vi "CAlex2_SetLegDH.vi"(8 "error in (no error)":errorcluster, 9 "End Effector Pos":T1={"Coord4"=[0.0, 0.0, 0.0, 1.0], "ID"=4}, 10 "ArmProperty":T2, 11 "CAlex2 in":refnum<class "CAlex2.lvclass">) -> (0 "error out":errorcluster, 3 "CAlex2 out":refnum<class "CAlex2.lvclass">)   [LabVIEW 2016, in "CAlex2.lvclass"]
uses:
  CAlex2.lvclass
  C:/Users/randh/Desktop/CABLE-LABVIEW/CALEX/CAlex2-controller/Classes/SerialChain/SerialChain.lvclass
  TypeDef/LowerBodyDim.ctl
  SerialChain/TypeDef/PointOnBody.ctl
  SerialChain/TypeDef/xyzO.ctl
  SerialChain/TypeDef/JointType.ctl
  SerialChain/SerialChain.lvclass
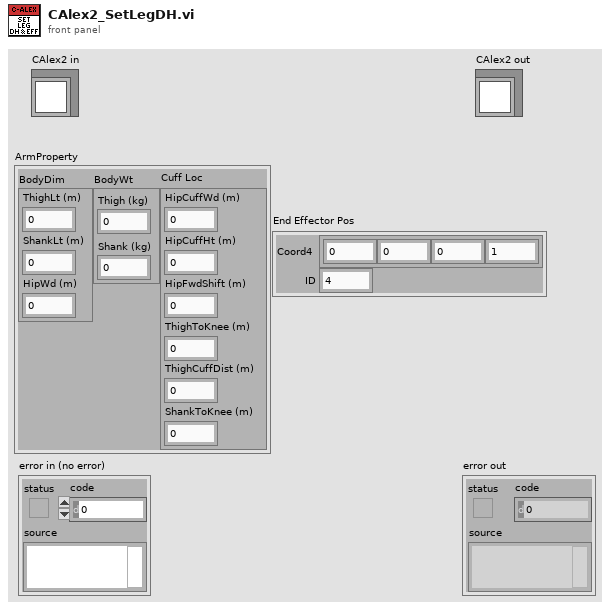
[diagram p1: front panel]
types:
  T1 = typedef "SerialChain.lvclass/PointOnBody.ctl" = cluster{"Coord4":dbl[], "ID":i32}
  T2 = typedef "CAlex2.lvclass/LowerBodyDim.ctl" = cluster{"BodyDim":cluster{"ThighLt (m)":dbl, "ShankLt (m)":dbl, "HipWd (m)":dbl}, "BodyWt":cluster{"Thigh (kg)":dbl, "Shank (kg)":dbl}, "Cuff Loc":cluster{"HipCuffWd (m)":dbl, "HipCuffHt (m)":dbl, "HipFwdShift (m)":dbl, "ThighToKnee (m)":dbl, "ThighCuffDist (m)":dbl, "ShankToKnee (m)":dbl}}
  T3 = typedef "SerialChain.lvclass/JointType.ctl" = enum16{"theta(hinge)", "alpha", "a", "d(slide)"}
  T4 = typedef "SerialChain.lvclass/xyzO.ctl" = enum16{"X", "Y", "Z", "O"}
  T5 = typedef "SerialChain.lvclass/DH_param.ctl" = cluster{"a":dbl, "d":dbl, "theta":dbl, "alpha":dbl, "JointType":T3}
  T6 = cluster{"DH Parameters":T5, "CoM_Pos":T1, "Mass(kg)":dbl}
  T7 = cluster{"DH Parameters":T5, "CoM_Pos":T1, "Mass(kg)":dbl}[]
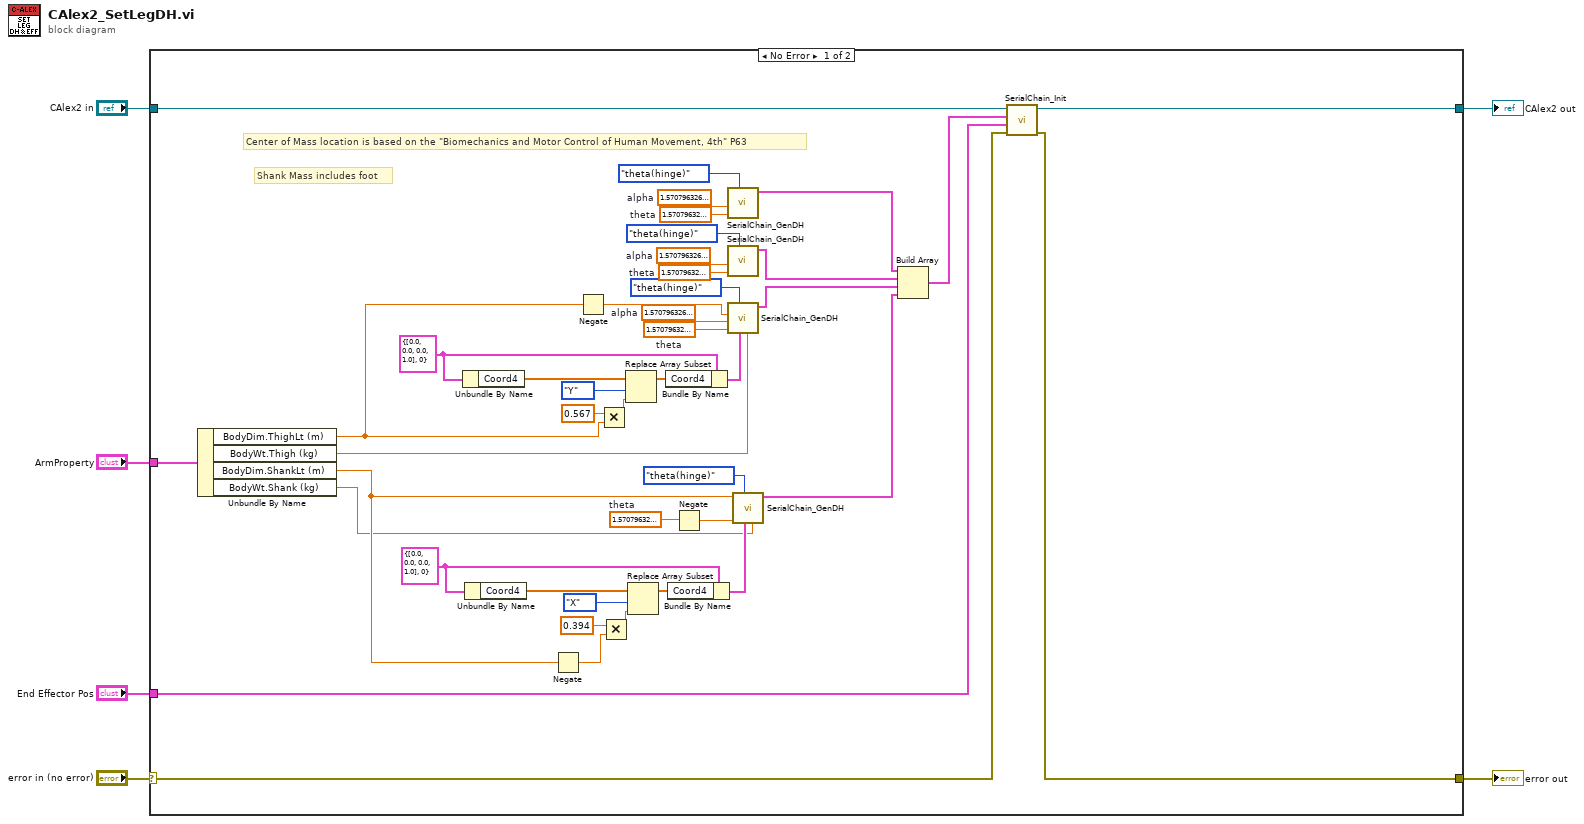
[diagram p0: block diagram]
diagram:
  n1 = case shown="No Error" "error in (no error)" {
    selector: "error in (no error)" -> [w17 w51]
    tunnel: [w8 w51] -> w5
    tunnel: [w7 w50] -> w3
    tunnel: "CAlex2 in" -> [w18 w50]
    tunnel: "ArmProperty" -> [w12 _]
    tunnel: "End Effector Pos" -> [w9 _]
    frame No Error {
      w21 = T1 {"Coord4"=[0.0, 0.0, 0.0, 1.0], "ID"=0} ("CoM_Pos")
      w31 = T1 {"Coord4"=[0.0, 0.0, 0.0, 1.0], "ID"=0} ("CoM_Pos")
      w38 = 1.5707963267948966  # theta
      w39 = 1.5707963267948966  # theta
      w40 = 1.5707963267948966  # theta
      w41 = 1.5707963267948966  # theta
      w48 = 1.5707963267948966  # alpha
      w42 = 1.5707963267948966  # alpha
      w49 = 1.5707963267948966  # alpha
      # "Shank Mass includes foot"
      # "Center of Mass location is based on the \"Biomechanics and Motor Control of Human Movement, 4th\" P63"
      n2 = Unbundle By Name(w12) -> ("BodyDim.ThighLt (m)"=w23:dbl, "BodyWt.Thigh (kg)"=w36:dbl, "BodyDim.ShankLt (m)"=w11:dbl, "BodyWt.Shank (kg)"=w10:dbl)
      n3 = Unbundle By Name(w31) -> ("Coord4"=w32:dbl[])
      n4 = Unbundle By Name(w21) -> ("Coord4"=w27:dbl[])
      n5 = Negate(x=w11) -> (-x=w19:dbl)
      n6 = Negate(x=w23) -> (-x=w22:dbl)
      n7 = Multiply(x=0.567, y=w23) -> (x*y=w33:dbl)
      n8 = Multiply(x=0.394, y=w19) -> (x*y=w26:dbl)
      n9 = Replace Array Subset(array=w32, new element=w33, index=xyzO."Y" ("XYZ")) -> (w30:dbl[])
      n10 = Replace Array Subset(array=w27, new element=w26, index=xyzO."X" ("XYZ")) -> (w28:dbl[])
      n11 = Bundle By Name(cluster=w31, "Coord4"=w30) -> (w29:T1)
      n12 = Bundle By Name(cluster=w21, "Coord4"=w28) -> (w20:T1)
      n13 = Negate(x=w38) -> (-x=w37:dbl)
      n14 = call "SerialChain_GenDH.vi"("JointType(hinge)"=JointType."theta(hinge)" ("JointType"), "theta(0)"=w41, "alpha(0)"=w49) -> ("DH Segment Cluster"=w47:T6)  [unwired: 8 in]
      n15 = call "SerialChain_GenDH.vi"("JointType(hinge)"=JointType."theta(hinge)" ("JointType"), "theta(0)"=w40, "alpha(0)"=w42) -> ("DH Segment Cluster"=w46:T6)  [unwired: 8 in]
      n16 = call "SerialChain_GenDH.vi"("Mass(kg)"=w36, "CoM Position (Origin)"=w29, "JointType(hinge)"=JointType."theta(hinge)" ("JointType"), "theta(0)"=w39, "alpha(0)"=w48, "d(0)"=w22) -> ("DH Segment Cluster"=w45:T6)  [unwired: 5 in]
      n17 = call "SerialChain_GenDH.vi"("Mass(kg)"=w10, "CoM Position (Origin)"=w20, "JointType(hinge)"=JointType."theta(hinge)" ("JointType"), "theta(0)"=w37, "a(0)"=w11) -> ("DH Segment Cluster"=w44:T6)  [unwired: 6 in]
      n18 = Build Array(w47, w46, w45, w44) -> (w43:T7)
      n19 = call "SerialChain_Init.vi"("error in (no error)"=w17, "End Effector Pos"=w9, "KnownDHVars"=w43, "SerialChain in"=w18) -> ("error out"=w8:errorcluster, "SerialChain out"=w7:refnum<class "CAlex2.lvclass">)  [unwired: 6 in]
    }
    frame Error {
    }
  }
  "error out" <- w5
  "CAlex2 out" <- w3
